vi "Test Executive.vi"(11 "Module Config":T30={"Name"="Test Executive", "Parent Q"=refnum, "Is Child?"=FALSE, "Index"=0, "Dirs"={"Root"=path "C:/MTE", "Config"=path "C:/MTE/Config", "Logs"=path "C:/MTE/Logs", "Reports"=path "C:/ATE/Reports", "App Data"=path "C:/ProgramData/Test Executive"}, "Simulate"=FALSE, "SimCtrl"=refnum}) -> ()   [LabVIEW 2018] (continued)
            n2238 = call <vilib>:"SeqMgr.Set Test Stop Criteria.vi"("Stop on Error"=w4705, "Stop on Fail"=w4706, "SeqMgr in"=w4734) -> ("SeqMgr out"=w4733:refnum<class "SeqMgr.lvclass">)  [unwired: 7 in, 1 out]
            n2239 = Build Array(w4712) -> (w4713:T31[])
            n2240 = Unbundle By Name(w4689) -> ("Opts.DisResults"=w4701:bool, "Opts.DispDetails"=w4699:bool)
            n2241 = call <vilib>:"File.Create Folder if Does Not Exist.vi"("Path"=w4698) -> ("Dup Path"=w4697:path)  [unwired: 8 in, 2 out]
            n2242 = To Variant(anything=w4713) -> (Variant=w4714:variant)
            n2243 = call <vilib>:"Q.Enqueue Task.vi"("Top of Q"=w4709, "Data1"=w4714, "Task Name"="Client - SW Items", "Q In"=w4700) -> ()  [unwired: 6 in, 2 out]
            n2244 = call <vilib>:"File.Delete Files and SubFolders in a Dir.vi"("Dir"=w4697) -> ("Dup Dir"=w4717:path)  [unwired: 9 in, 1 out]
            n2245 = Path To String(path=w4717) -> (string=w4716:string)
            n2246 = local read "Start Time"() -> (w4669:timestamp)
            n2247 = property on="Mode" class="Ring (strict)"() -> ("RingText.Text"=w4682:string)  [unwired: 2 in, 2 out]
            n2248 = local read "Default Timeout (s)"() -> (w4684:dbl)
            n2249 = local read "SN"() -> (w4740:string)
            n2250 = Bundle By Name(cluster=w4689, "DisableResults"=w4701) -> (w4665:T73)
            n2251 = Format Date/Time String(time format string (%c)="%Y_%m_%d") -> (date/time string=w4674:string)  [unwired: 2 in]
            n2252 = Select(t=1, s=w4699, f=0) -> (s? t:f=w4667:i32)
            n2253 = Format Date/Time String(time format string (%c)="%Y%m%d_%H%M%S", seconds (now)=w4669) -> (date/time string=w4672:string)  [unwired: 1 in]
            n2254 = local write "Test Status Tab Sel"(w4667) -> ()
            n2255 = local write "Test Status Tab"(w4667) -> ()
            n2256 = Number To Fractional String(number=w4684) -> (F-format string=w4742:string)  [unwired: 3 in]
            n2257 = Build Array("Mode", w4682) -> (w4680:string[])
            n2258 = Build Array("SN", w4740) -> (w4741:string[])
            n2259 = Build Array("DirSeq", w4685) -> (w4692:string[])
            n2260 = Build Array("DirCfg", w4686) -> (w4691:string[])
            n2261 = Build Array("ReportFileDir", w4716) -> (w4715:string[])
            n2262 = Build Array("Date", w4674) -> (w4676:string[])
            n2263 = Build Array("UUTDir", "") -> (w4661:string[])
            n2264 = Build Array("StartTime", w4672) -> (w4668:string[])
            n2265 = Build Array("DelaySecs", w4742) -> (w4681:string[])
            n2266 = Build Array (concatenate)(w4681, w4680, w4741, string[][] [["Failing", "0"], ["Error", "0"], ["Abort", "0"]], w4668, w4676, w4661, w4715, w4692, w4691) -> (w4735:string[][])
            n2267 = Unbundle By Name(w4665) -> ("Lists.ProcessStep"=w4663:string, "Lists.Product"=w4664:string)
            n2268 = call <vilib>:"SeqMgr.Variables - Add, Replace.vi"("Name, Value"=w4735, "Init"=TRUE, "SeqMgr in"=w4733) -> ("SeqMgr out"=w4736:refnum<class "SeqMgr.lvclass">)  [unwired: 7 in, 1 out]
            n2269 = invoke on="OperNo" class="Bool" method="Reinit To Default"() -> ()  [unwired: 3 in, 3 out]
            n2270 = invoke on="OperOK" class="Bool" method="Reinit To Default"() -> ()  [unwired: 3 in, 3 out]
            n2271 = invoke on="Prompt2_OK" class="Bool" method="Reinit To Default"() -> ()  [unwired: 3 in, 3 out]
            n2272 = call "Step Counter.Step Count Controller.vi"("Step Action"=Step_Counter.Action."Init") -> ("Step State Out"=w4732:T72)  [unwired: 8 in, 2 out]
            n2273 = Bundle By Name(cluster=w4665, "RptHdr.Test Run.ProcessStep"=w4663, "RptUUT.UUTInfo.Product"=w4664, "TimeOut(s)"="Default Timeout (s)", "SeqMgr"=w4736, "SectCtr"=w4732, "TestCanceled"=FALSE, "Data"=cluster{"FileObjs":T29[], "Meas":T38[]} {"FileObjs"=[], "Meas"=[]}) -> (w4730:T73)
            n2274 = invoke on="OperPict" class="Pict" method="Reinit To Default"() -> ()  [unwired: 3 in, 3 out]
            n2275 = property on="Operator" class="Str"("DisabledEnum"=w4724, "Text.BGColor"=w4723) -> ()  [unwired: 2 in, 2 out]
            n2276 = property on="SN" class="Str"("DisabledEnum"=w4724, "Text.BGColor"=w4723) -> ()  [unwired: 2 in, 2 out]
            n2277 = property on="Show Only Failures" class="Bool (strict)"("DisabledEnum"=T36."Disabled and Grayed Out" ("Disabled"), "Value"=FALSE ("Show Only Failures")) -> ()  [unwired: 2 in, 2 out]
            n2278 = property on="Results Table" class="Arr (strict)"("Index Values"=u32[] [0]) -> ()  [unwired: 2 in, 2 out]
          }
          frame "Test Running" {
            n2279 = Unbundle By Name(w4747) -> ("SeqMgr"=w4774:refnum<class "SeqMgr.lvclass">, "ResultState"=w4770:T63, "ResultError"=w4769:errorcluster)
            n2280 = call <vilib>:"Q.Enqueue Seq.vi"("Seq Task Name"="List Vars", "Q In"=w4751) -> ("Q Out"=w4749:refnum<queue>)  [unwired: 8 in, 1 out]
            n2281 = call <vilib>:"SeqMgr.Update Progress.vi"("error in"=w4769, "Result Info"=w4770, "SeqMgr in"=w4774) -> ("Result Info Out"=w4767:T63, "Test State"=w4771:enum32{"Idle", "Running", "Completed"}, "SeqMgr out"=w4759:refnum<class "SeqMgr.lvclass">, "New Step"=w4765:string[], "Canceled"=w4766:bool, "StepCnt"=w4748:i32)  [unwired: 2 in, 1 out]
            "Step" <- w4765
            "StepCnt" <- w4748
            n2282 = Delete From Array(array=w4765, index=0) -> (deleted portion=w4773:string, array with subset deleted=w4768:string[])  [unwired: 1 in]
            n2283 = case shown="\"Completed\"" w4771 {
              tunnel: w4773 -> [_ w4792 _]
              tunnel: w4749 -> [_ w4788 w4822]
              tunnel: ["Idle" w4790 w4826] -> w4763
              tunnel: w4767 -> [w4775 w4779 w4825]
              tunnel: w4768 -> [_ w4785 _]
              tunnel: [Event_Log.Notification_Type."Normal" ("Type") Event_Log.Notification_Type."Normal" ("Type") w4824] -> w4762
              tunnel: [Event_Log.Log_Level."Debug0" ("Level") Event_Log.Log_Level."Debug0" ("Level") Event_Log.Log_Level."Normal" ("Level")] -> w4761
              tunnel: w4748 -> [_ w4780 _]
              tunnel: w4747 -> [_ _ w4820]
              tunnel: w4746 -> [_ _ w4819]
              tunnel: [w4775 w4779 w4818] -> w4745
              frame "Idle", Default {
                # "Do Nothing"
              }
              frame "Running" {
                n2284 = To Lower Case(string=w4792) -> (all lower case string=w4794:string)
                n2285 = local read "Pause"() -> (w4791:bool)
                n2286 = Array To Spreadsheet String(delimiter (Tab)=",", array=w4785, 3:"" ("format string")) -> (spreadsheet string=w4782:string)
                n2287 = Match Pattern(string=w4794, regular expression="^sta\\.") -> (after substring=w4789:string, offset past match=w4793:i32)  [unwired: 1 in, 2 out]
                n2288 = call <vilib>:"Trim Whitespace.vi"("string"=w4782) -> ("trimmed string"=w4781:string)  [unwired: 1 in]
                n2289 = case shown="True" w4791 {
                  frame False {
                  }
                  frame True {
                    n2290 = while {
                      stop <- w4800 stop-if-true
                      n2291 = Not(x="Pause") -> (.not. x?=w4798:bool)
                      n2292 = Or(x="Inc Step", y=w4798) -> (x .or. y?=w4800:bool)
                      n2293 = Wait (ms)(milliseconds to wait=u32 100) -> ()  [unwired: 1 out]
                    }
                  }
                }
                n2294 = case shown="0, Default" w4793 {
                  tunnel: w4792 -> [w4807 w4811]
                  tunnel: w4785 -> [w4809 w4817]
                  tunnel: w4789 -> [_ _]
                  tunnel: w4788 -> [w4803 w4813]
                  frame 0, Default {
                    # "The RTN will \nCall the Test Running\nState"
                    n2295 = String Subset(string=w4807, offset (0)=4) -> (substring=w4805:string)  [unwired: 1 in]
                    n2296 = Build Array (concatenate)(w4805, w4809) -> (w4808:string[])
                    n2297 = To Variant(anything=w4808) -> (Variant=w4802:variant)
                    n2298 = call <vilib>:"Q.Enqueue Task.vi"("Data1"=w4802, "Task Name"="StaCmd", "Q In"=w4803) -> ()  [unwired: 7 in, 2 out]
                  }
                  frame -1 {
                    n2299 = To Variant(anything=w4817) -> (Variant=w4814:variant)
                    n2300 = To Variant(anything=w4811) -> (Variant=w4812:variant)
                    n2301 = call <vilib>:"Q.Enqueue Task.vi"("Data2"=w4812, "Data1"=w4814, "Task Name"="SeqCmd", "Q In"=w4813) -> ("Q Out"=w4815:refnum<queue>)  [unwired: 6 in, 1 out]
                    n2302 = call <vilib>:"Q.Enqueue Seq.vi"("Seq Task Name"="Test Running", "Q In"=w4815) -> ()  [unwired: 8 in, 2 out]
                  }
                }
                n2303 = Format Into String(format string="Test Step: Cnt_%d %s, %s", w4780, w4792, w4781) -> (resulting string=w4790:string)  [unwired: 2 in, 1 out]
              }
              frame "Completed" {
                n2304 = Flush Queue(queue=w4822) -> (queue out=w4821:refnum<queue>)  [unwired: 1 in, 2 out]
                n2305 = Unbundle By Name(w4825) -> ("State"=w4827:T1)
                n2306 = call <vilib>:"Q.Enqueue Seq.vi"("Seq Task Name"="Test Completed", "Q In"=w4821) -> ()  [unwired: 8 in, 2 out]
                n2307 = case shown="\"None\", Default" w4827 {
                  selector: w4827 -> [w4832 w4838 _ _]
                  tunnel: [w4831 w4836 w4848 w4857] -> w4826
                  tunnel: w4825 -> [w4829 w4834 w4841 w4855]
                  tunnel: [Event_Log.Notification_Type."Normal" ("Type") Event_Log.Notification_Type."Success" ("Type") Event_Log.Notification_Type."Error" ("Type") Event_Log.Notification_Type."Error" ("Type")] -> w4824
                  tunnel: w4820 -> [_ _ w4845 _]
                  tunnel: w4819 -> [_ _ w4844 _]
                  tunnel: [w4829 w4834 w4839 w4855] -> w4818
                  frame "None", Default {
                    n2308 = Format Into String(format string="Test Completed: %s" ("Seq Task Name"), w4832) -> (resulting string=w4831:string)  [unwired: 2 in, 1 out]
                  }
                  frame "Passing", "PASS" {
                    n2309 = Format Into String(format string="Test Completed: %s" ("Seq Task Name"), w4838) -> (resulting string=w4836:string)  [unwired: 2 in, 1 out]
                  }
                  frame "Failing", "FAIL" {
                    n2310 = Unbundle By Name(w4844) -> ("Cfg.Dirs.Config"=w4843:path)
                    n2311 = Unbundle By Name(w4845) -> ("Data.Meas"=w4846:T38[])
                    n2312 = call "Results.Evaluate Overall Result Based on Failure Priority.vi"("ConfigDir"=w4843, "Meas"=w4846) -> ("Change"=w4842:bool, "Result Info"=w4840:T63)  [unwired: 8 in]
                    n2313 = case shown="True" w4842 {
                      tunnel: w4841 -> [w4853 _]
                      tunnel: w4840 -> [_ w4854]
                      tunnel: [w4853 w4854] -> w4839
                      frame False {
                      }
                      frame True {
                      }
                    }
                    n2314 = Unbundle By Name(w4839) -> ("State"=w4851:T1, "Code"=w4850:i32, "Description"=w4849:string)
                    n2315 = Format Into String(format string="Test Completed: %s, %d, %s" ("Seq Task Name"), w4851, w4850, w4849) -> (resulting string=w4848:string)  [unwired: 2 in, 1 out]
                  }
                  frame "ERROR" {
                    n2316 = Unbundle By Name(w4855) -> ("State"=w4860:T1, "Code"=w4859:i32, "Description"=w4858:string)
                    n2317 = Format Into String(format string="Test Completed: %s, %d, %s" ("Seq Task Name"), w4860, w4859, w4858) -> (resulting string=w4857:string)  [unwired: 2 in, 1 out]
                  }
                }
              }
            }
            n2318 = Bundle By Name(cluster=w4747, "TestCanceled"=w4766, "SeqMgr"=w4759) -> (w4744:T73)
            n2319 = call <vilib>:"SeqMgr.Variables - Get.vi"("SeqMgr in"=w4759) -> ("Vars"=w4758:variant)  [unwired: 8 in, 2 out]
            n2320 = Get Variant Attribute(Variant=w4758) -> (names=w4754:string[], values=w4757:variant[])  [unwired: 3 in, 2 out]
            n2321 = Variant To Data(type=string[] [], Variant=w4757) -> (data=w4755:string[])  [unwired: 1 in, 1 out]
            n2322 = Build Array(w4754, w4755) -> (w4752:string[][])
            n2323 = Unbundle By Name(w4746) -> ("Log"=w4764:refnum<class "Event Notification.lvclass">)
            n2324 = Transpose 2D Array(2D array=w4752) -> (transposed array=w4753:string[][])
            n2325 = local write "Variables"(w4753) -> ()
            n2326 = call <vilib>:"Event Notification.Status Message with Error In.vi"("Log"=TRUE, "Level"=w4761, "Type"=w4762, "Message"=w4763, "Event Notification in"=w4764) -> ()  [unwired: 7 in]
            n2327 = Bundle By Name(cluster=w4744, "ResultState"=w4745) -> (w4743:T73)
          }
          frame "List Vars" {
            n2328 = Unbundle By Name(w4863) -> ("Lists.ReqVars"=w4862:bool)
            "Var Subscribe" <- w4862
            n2329 = Unbundle By Name(w4863) -> ("SeqMgr"=w4871:refnum<class "SeqMgr.lvclass">)
            n2330 = call <vilib>:"SeqMgr.Variables - Get.vi"("SeqMgr in"=w4871) -> ("Vars"=w4864:variant)  [unwired: 8 in, 2 out]
            n2331 = case shown="True" w4862 {
              tunnel: w4863 -> [_ w4876]
              tunnel: w4864 -> [_ w4873]
              frame False {
              }
              frame True {
                n2332 = Unbundle By Name(w4876) -> ("StaApp"=w4874:string)
                n2333 = call <vilib>:"Q.Enqueue Task.vi"("Data1"=w4873, "Q Name"=w4874, "Task Name"="Test Vars") -> ()  [unwired: 7 in, 2 out]
              }
            }
            n2334 = Get Variant Attribute(Variant=w4864) -> (names=w4870:string[], values=w4869:variant[])  [unwired: 3 in, 2 out]
            n2335 = Variant To Data(type=string[] [], Variant=w4869) -> (data=w4867:string[])  [unwired: 1 in, 1 out]
            n2336 = Build Array(w4870, w4867) -> (w4866:string[][])
            n2337 = Transpose 2D Array(2D array=w4866) -> (transposed array=→"Variables":string[][])
          }
          frame "Abort", "Test Abort" {
            n2338 = Unbundle By Name(w4879) -> ()  [unwired: 1 out]
            n2339 = local read "Test State"() -> (w4887:enum32{"Idle", "Running", "Completed"})
            n2340 = case shown="\"Running\"" w4887 {
              tunnel: w4879 -> [_ w4900]
              tunnel: w4880 -> [_ w4897]
              frame "Idle", Default {
              }
              frame "Running" {
                # "Return to Test Running to process the Abort"
                # "Delete timeout for \ncurrent function"
                n2341 = Unbundle By Name(w4900) -> ("Funct.Name"=w4894:string, "StaApp"=w4899:string)
                n2342 = call <vilib>:"Q.Enqueue Seq.vi"("Top of Q"=TRUE, "Seq Task Name"="Test Running", "Q In"=w4897) -> ("Q Out"=w4893:refnum<queue>)  [unwired: 7 in, 1 out]
                n2343 = local write "Abort Flag"(TRUE ("Repeat Seq")) -> ()
                n2344 = call <vilib>:"Q.Enqueue Task.vi"("Top of Q"=TRUE, "Q Name"=w4899, "Task Name"="Abort" ("Seq Task Name")) -> ()  [unwired: 7 in, 2 out]
                n2345 = call <vilib>:"Scheduler.Delete Task.vi"("Sched Name"=w4894, "Q In"=w4893) -> ()  [unwired: 8 in, 2 out]
                n2346 = for {
                  N: 5 -> [_]
                  n2347 = call "Abort.Send Abort or Done Notificaiton.vi"("Abort(T)/Done(F)"=TRUE) -> ()  [unwired: 10 in, 1 out]
                  n2348 = Wait (ms)(milliseconds to wait=u32 10) -> ()  [unwired: 1 out]
                }
              }
            }
            n2349 = local write "Repeat Seq"(FALSE ("Repeat Seq")) -> ()
            n2350 = Bundle By Name(cluster=w4879, "Funct.Seq"=0, "Funct.Name"="", "ResultState.State"=SeqMgr.Result_State_Enum."ABORT" ("State"), "ResultState.Code"=-1 ("Code"), "ResultState.Description"="Test aborted by operator.", "Repeat(s)"=-1.0) -> (w4883:T73)
            n2351 = Unbundle By Name(w4883) -> ("SeqMgr"=w4886:refnum<class "SeqMgr.lvclass">)
            n2352 = call <vilib>:"SeqMgr.Variables - Add, Replace.vi"("Name, Value"=string[][] [["Abort", "1"]] ("appended array"), "SeqMgr in"=w4886) -> ("SeqMgr out"=w4885:refnum<class "SeqMgr.lvclass">)  [unwired: 8 in, 1 out]
            n2353 = Bundle By Name(cluster=w4883, "SeqMgr"=w4885) -> (w4882:T73)
          }
          frame "Test Completed" {
            # "Clear Abort"
            n2354 = Unbundle By Name(w4915) -> ("Repeat(s)"=w4943:dbl, "Opts.NotResetSN"=w4941:bool)
            n2355 = Unbundle By Name(w4915) -> ("ResultState"=w4914:T63)
            n2356 = Unbundle By Name(w4915) -> ("Opts.DispDetails"=w4945:bool, "Opts.DisResults"=w4912:bool, "Opts.DisMetrics"=w4927:bool, "TestCanceled"=w4911:bool)
            n2357 = local write "Funct Tab"(0) -> ()
            n2358 = Unbundle By Name(w4915) -> ("StaApp"=w4918:string)
            n2359 = Unbundle By Name(w4915) -> ("PreTestCk.SNErr"=w4921:bool, "PreTestCk.NoSN"=w4924:bool, "PreTestCk.DefaultSN"=w4923:string)
            n2360 = To Variant(anything=w4914) -> (Variant=w4919:variant)
            n2361 = call <vilib>:"Q.Enqueue Task.vi"("Top of Q"=TRUE, "Data1"=w4919, "Q Name"=w4918, "Task Name"="Test Status") -> ()  [unwired: 6 in, 2 out]
            n2362 = Greater Or Equal To 0?(x=w4943) -> (x >= 0?=w4942:bool)
            n2363 = call <vilib>:"Q.Enqueue Task.vi"("Task Name"="StaTest End", "Q In"=w4934) -> ("Q Out"=w4935:refnum<queue>)  [unwired: 8 in, 1 out]
            n2364 = Or(x=w4942, y=w4941) -> (x .or. y?=w4922:bool)
            n2365 = Unbundle By Name(w4915) -> ("RptHdr.Station.SW_Config.SW_Item"=→"SW Items":T31[], "RptHdr.Test Sequence.Config.Config_Item"=→"Seq Setup":cluster{"Name":string, "Value":string}[])
            n2366 = Or(x=w4927, y=w4911) -> (x .or. y?=w4951:bool)
            n2367 = Or(x=w4922, y=w4921) -> (x .or. y?=w4920:bool)
            n2368 = case shown="True" w4945 {
              tunnel: [u32 0 w4979] -> w4913
              frame False {
              }
              frame True {
                n2369 = local read "Test Status Tab"() -> (w4975:T6)
                n2370 = To Unsigned Long Integer(number=w4975) -> (unsigned 32bit integer=w4976:u32)
                n2371 = In Range and Coerce(upper limit=u32 1, x=w4976, lower limit=u32 0) -> (coerced(x)=w4979:u32)  [unwired: 1 out]
              }
            }
            n2372 = case shown="False" w4951 {
              tunnel: w4935 -> [w4988 w4989]
              tunnel: [w4987 w4989] -> w4907
              tunnel: "Test Metrics - Add" -> [w4986 _]
              frame False {
                n2373 = call <vilib>:"Q.Enqueue Task.vi"("Task Name"=w4986, "Q In"=w4988) -> ("Q Out"=w4987:refnum<queue>)  [unwired: 8 in, 1 out]
              }
              frame True {
              }
            }
            n2374 = case shown="False" w4920 {
              tunnel: w4924 -> [w4983 _]
              tunnel: w4923 -> [w4982 _]
              frame False {
                n2375 = case shown="True" w4983 {
                  tunnel: w4982 -> [_ w4985]
                  frame False {
                    n2376 = invoke on="SN" class="Str" method="Reinit To Default"() -> ()  [unwired: 3 in, 3 out]
                    n2377 = property on="SN" class="Str"("Text.FontSize"=u32 20 ("F1")) -> ()  [unwired: 2 in, 2 out]
                  }
                  frame True {
                    n2378 = local write "SN"(w4985) -> ()
                  }
                }
              }
              frame True {
              }
            }
            n2379 = Or(x=w4912, y=w4911) -> (x .or. y?=w4910:bool)
            n2380 = call <vilib>:"Q.Enqueue Task.vi"("Task Name"="Result Comment", "Q In"=w4907) -> ("Q Out"=w4906:refnum<queue>)  [unwired: 8 in, 1 out]
            n2381 = local read "Result Status"() -> (→"Result Status 2":T2)
            n2382 = property on="SN" class="Str"("Key Focus"=TRUE) -> ()  [unwired: 2 in, 2 out]
            n2383 = case shown="False" w4910 {
              tunnel: [w4999 w5001] -> w4967
              tunnel: w4906 -> [w4999 w5000]
              frame True {
              }
              frame False {
                n2384 = call <vilib>:"Q.Enqueue Task.vi"("Task Name"="Result - Reports", "Q In"=w5000) -> ("Q Out"=w5001:refnum<queue>)  [unwired: 8 in, 1 out]
              }
            }
            n2385 = local write "Test Status Tab"(w4913) -> ()
            n2386 = local write "Test Status Tab Sel"(w4913) -> ()
            n2387 = call "Abort.Send Abort or Done Notificaiton.vi"("Abort(T)/Done(F)"=FALSE) -> ()  [unwired: 10 in, 1 out]
            n2388 = property on="State" class="Enum (strict)"() -> (error out=w4955:errorcluster, "RingText.BGColor"=w4954:u32)  [unwired: 2 in, 1 out]
            n2389 = To Variant(anything=FALSE) -> (Variant=w4968:variant)
            n2390 = Unbundle By Name(w4915) -> ("Opts.SetOpts"=w4926:bool)
            n2391 = call <vilib>:"Q.Enqueue App.vi"("Data1"=w4968, "Task Name"="Lock Test Controls", "Q In"=w4967) -> ("Q Out"=w4938:refnum<queue>)  [unwired: 7 in, 1 out]
            n2392 = Unbundle By Name(w4915) -> ("Repeat(s)"=w4930:dbl)
            n2393 = call <vilib>:"Q.Enqueue Task.vi"("Task Name"="Sta Notify", "Q In"=w4938) -> ("Q Out"=w4939:refnum<queue>)  [unwired: 8 in, 1 out]
            n2394 = property on="State" class="Enum (strict)"(error in=w4955, "RingText.BGColor"=w4954) -> ()  [unwired: 1 in, 2 out]
            n2395 = local read "Duration(s)"() -> (w4963:dbl)
            n2396 = Greater Or Equal To 0?(x=w4930) -> (x >= 0?=w4932:bool)
            n2397 = case shown="False" w4926 {
              frame False {
                n2398 = local write "Funct Tab"(u32 0) -> ()
              }
              frame True {
              }
            }
            n2399 = To Variant(anything="Init") -> (Variant=w4950:variant)
            n2400 = call <vilib>:"Q.Enqueue Seq.vi"("Data1"=w4950, "Seq Task Name"="Test Idle", "Q In"=w4939) -> ("Q Out"=w4937:refnum<queue>)  [unwired: 7 in, 1 out]
            n2401 = property on="Inc Step" class="Bool"("DisabledEnum"=T36."Disabled and Grayed Out" ("Disabled")) -> ()  [unwired: 2 in, 2 out]
            n2402 = property on="Step Run" class="Bool"("DisabledEnum"=T36."Disabled and Grayed Out" ("Disabled")) -> ()  [unwired: 2 in, 2 out]
            n2403 = case shown="True" "Repeat Seq" {
              selector: "Repeat Seq" -> [_ w4973]
              tunnel: w4932 -> [w4971 _]
              tunnel: [w4971 w4973] -> w4931
              tunnel: w4930 -> [w4970 _]
              tunnel: [w4970 w4972] -> w4929
              tunnel: "RepeatInt(s)" -> [_ w4972]
              frame False {
              }
              frame True {
              }
            }
            n2404 = local read "SN Rslt"() -> (w4944:string)
            n2405 = stacked-sequence {
              frame #0 {
                n2406 = local write "Test Ctrl Tab"(enum32{"Idle", "Running", "Completed"}."Idle" ("Test Ctrl Tab")) -> ()
              }
              frame #1 {
                n2407 = property on="Start" class="Bool"("Key Focus"=TRUE) -> ()  [unwired: 2 in, 2 out]
              }
            }
            n2408 = Bundle By Name(cluster=w4915, "RptHdr.Test Run.Duration(s)"=w4963) -> (w4964:T73)
            n2409 = case shown="True" w4931 {
              tunnel: "Repeat Sequence" ("Sched Name") -> [_ w4998]
              tunnel: w4929 -> [_ w4997]
              tunnel: w4937 -> [_ w4996]
              tunnel: w4944 -> [_ w4990]
              frame False {
              }
              frame True {
                w4992 = TRUE ("Visible")
                n2410 = To Variant(anything=w4990) -> (Variant=w4991:variant)
                n2411 = call <vilib>:"Scheduler.AddTask.vi"("Data1"=w4991, "Interval(s)"=w4997, "Task Name"=w4998, "Sched Name"=w4998, "Q In"=w4996) -> ("Q Out"=w4995:refnum<queue>)  [unwired: 5 in, 1 out]
                n2412 = property on="Repeat Notificaiton" class="Str"("Visible"=w4992) -> ()  [unwired: 2 in, 2 out]
                n2413 = property on="Kill AutoLnch" class="Bool"("Visible"=w4992) -> ()  [unwired: 2 in, 2 out]
                n2414 = call <vilib>:"Q.Enqueue Task.vi"("Top of Q"=TRUE, "Task Name"="Repeat Notification" ("Sched Name"), "Q In"=w4995) -> ()  [unwired: 7 in, 2 out]
              }
            }
            n2415 = property on="Show Only Failures" class="Bool (strict)"("DisabledEnum"=T36."Enabled" ("Disabled")) -> ()  [unwired: 2 in, 2 out]
            "Test State" <- enum32{"Idle", "Running", "Completed"}."Completed" ("Test State")
          }
          frame "Test Reset" {
            w5008 = picture data[5B] ("Rigth Image")
            w5015 = FALSE
            w5028 = u32 16448250
            w5031 = T36."Enabled" ("Disabled")
            # "Clear Abort Notificaiton"
            # "Clear data to prepare for a new test"
            n2416 = Obtain Notifier(name (unnamed)="Abort", notification data type=w5015) -> (notifier out=w5019:refnum<notifier>, error out=w5018:errorcluster)  [unwired: 2 in, 1 out]
            n2417 = call <vilib>:"Scheduler.Delete Task.vi"("Sched Name"="Repeat Sequence", "Q In"=w5034) -> ("Q Out"=w5012:refnum<queue>)  [unwired: 8 in, 1 out]
            n2418 = invoke on="SN Rslt" class="Str" method="Reinit To Default"() -> ()  [unwired: 3 in, 3 out]
            n2419 = Unbundle By Name(w5027) -> ("Log"=w5026:refnum<class "Event Notification.lvclass">)
            n2420 = Send Notification(notification=w5015, notifier=w5019, error in (no error)=w5018) -> (notifier out=w5016:refnum<notifier>, error out=w5017:errorcluster)
            n2421 = call <vilib>:"Q.Enqueue Task.vi"("Task Name"="Sta Test Reset", "Q In"=w5012) -> ("Q Out"=w5011:refnum<queue>)  [unwired: 8 in, 1 out]
            n2422 = call <vilib>:"Event Notification.Status Message.vi"("Display"=TRUE, "Level"=Event_Log.Log_Level."Normal", "Message"="Idle", "Event Notification in"=w5026) -> ()  [unwired: 8 in]
            n2423 = Release Notifier(notifier=w5016, force destroy? (F)=TRUE, error in (no error)=w5017) -> ()  [unwired: 3 out]
            n2424 = To Variant(anything="Init") -> (Variant=w5040:variant)
            n2425 = call <vilib>:"Q.Enqueue Seq.vi"("Data1"=w5040, "Seq Task Name"="Test Idle", "Q In"=w5011) -> ()  [unwired: 7 in, 2 out]
            n2426 = property on="Kill AutoLnch" class="Bool"("Visible"=FALSE) -> ()  [unwired: 2 in, 2 out]
            n2427 = property on="Repeat Notificaiton" class="Str"("Visible"=FALSE) -> ()  [unwired: 2 in, 2 out]
            n2428 = Unbundle By Name(w5007) -> ("SeqMgr"=w5044:refnum<class "SeqMgr.lvclass">, "Opts.NotResetSN"=w5020:bool, "Repeat(s)"=w5022:dbl)
            n2429 = local write "Test State"(enum32{"Idle", "Running", "Completed"}."Idle" ("Test State")) -> ()
            n2430 = invoke on="Duration(HH:MM:SS)" class="Str" method="Reinit To Default"() -> ()  [unwired: 3 in, 3 out]
            n2431 = Unbundle By Name(w5007) -> ("PreTestCk.NoSN"=w5006:bool, "PreTestCk.DefaultSN"=w5005:string, "PreTestCk.SeqEn"=w5003:T36)
            n2432 = Greater Or Equal To 0?(x=w5022) -> (x >= 0?=w5023:bool)
            n2433 = property on="SN" class="Str"("Key Focus"=TRUE) -> ()  [unwired: 2 in, 2 out]
            n2434 = Or(x=w5020, y=w5023) -> (x .or. y?=w5021:bool)
            n2435 = case shown="False" w5021 {
              tunnel: w5006 -> [w5049 _]
              tunnel: w5005 -> [w5048 _]
              frame False {
                n2436 = case shown="True" w5049 {
                  tunnel: w5048 -> [_ w5051]
                  frame False {
                    n2437 = invoke on="SN" class="Str" method="Reinit To Default"() -> ()  [unwired: 3 in, 3 out]
                    n2438 = property on="SN" class="Str"("Text.FontSize"=u32 20 ("F1")) -> ()  [unwired: 2 in, 2 out]
                  }
                  frame True {
                    n2439 = local write "SN"(w5051) -> ()
                  }
                }
              }
              frame True {
              }
            }
            n2440 = property on="Operator" class="Str"("DisabledEnum"=w5031, "Text.BGColor"=w5028) -> ()  [unwired: 2 in, 2 out]
            n2441 = call <vilib>:"SeqMgr.Test Reset.vi"("SeqMgr in"=w5044) -> ("SeqMgr out"=w5045:refnum<class "SeqMgr.lvclass">)  [unwired: 9 in, 1 out]
            n2442 = property on="SN" class="Str"("DisabledEnum"=w5031, "Text.BGColor"=w5028) -> ()  [unwired: 2 in, 2 out]
            n2443 = property on="Sequence" class="Ring (strict)"("DisabledEnum"=w5003) -> ()  [unwired: 2 in, 2 out]
            n2444 = property on="Results Table" class="Arr (strict)"("Index Values"=u32[] [0]) -> ()  [unwired: 2 in, 2 out]
            n2445 = Bundle By Name(cluster=w5007, "SeqMgr"=w5045) -> (w5043:T73)
            n2446 = invoke on="OperPrompt" class="Str" method="Reinit To Default"() -> ()  [unwired: 3 in, 3 out]
            n2447 = invoke on="Abort Flag" class="Bool (strict)" method="Reinit To Default"() -> ()  [unwired: 3 in, 3 out]
            n2448 = invoke on="Results Table" class="Arr (strict)" method="Reinit To Default"() -> ()  [unwired: 3 in, 3 out]
            n2449 = invoke on="OperPict" class="Pict" method="Reinit To Default"() -> ()  [unwired: 3 in, 3 out]
            n2450 = invoke on="Variables" class="Arr (strict)" method="Reinit To Default"() -> ()  [unwired: 3 in, 3 out]
            n2451 = invoke on="OperNo" class="Bool" method="Reinit To Default"() -> ()  [unwired: 3 in, 3 out]
            n2452 = invoke on="OperOK" class="Bool" method="Reinit To Default"() -> ()  [unwired: 3 in, 3 out]
            n2453 = invoke on="Prompt2_OK" class="Bool" method="Reinit To Default"() -> ()  [unwired: 3 in, 3 out]
            n2454 = invoke on="Progress 2" class="Slide (strict)" method="Reinit To Default"() -> ()  [unwired: 3 in, 3 out]
            n2455 = Bundle By Name(cluster=w5043, "RptHdr.Test Run"=T48 {"Operator"="", "Start Time"=timestamp(0 s since 1904-01-01), "Duration(s)"=0.0, "Mode"="", "Comment"="", "ProcessStep"=""} ("RptHdrInfo.Test Run"), "RptHdr.Test Sequence"=T49 {"Name"="", "Config"={"Config_Item"=[]}} ("RptHdrInfo.Test Sequence"), "RptUUT"=T50 {"Position"="", "Result"={"Result"=enum."Pass", "Code"=0, "Description"=""}, "Measurements"={"Measurement"=[]}, "UUTInfo"={"Product"="", "Desc"="", "PN"="", "SN"="", "Lot"="", "DateCode"="", "AltID"="", "Revision"="", "Properties"={"Property"=[]}}} ("RptUUTInfo"), "Data"=cluster{"FileObjs":T29[], "Meas":T38[]} {"FileObjs"=[], "Meas"=[]}) -> (w5046:T73)
            n2456 = local write "Rigth Image"(w5008) -> ()
            n2457 = local write "Left Image"(w5008) -> ()
            n2458 = invoke on="UUT Properties" class="Arr (strict)" method="Reinit To Default"() -> ()  [unwired: 3 in, 3 out]
            n2459 = invoke on="File Data Objs" class="Arr (strict)" method="Reinit To Default"() -> ()  [unwired: 3 in, 3 out]
            n2460 = invoke on="SeqPN" class="Str" method="Reinit To Default"() -> ()  [unwired: 3 in, 3 out]
            n2461 = invoke on="SeqVer" class="Str" method="Reinit To Default"() -> ()  [unwired: 3 in, 3 out]
            n2462 = invoke on="Seq Setup" class="Arr (strict)" method="Reinit To Default"() -> ()  [unwired: 3 in, 3 out]
            n2463 = invoke on="SeqName" class="Str" method="Reinit To Default"() -> ()  [unwired: 3 in, 3 out]
            "Test Ctrl Tab" <- enum32{"Idle", "Running", "Completed"}."Idle" ("Test Ctrl Tab")
          }
        }
      }
      frame "Function" {
        n2464 = case shown="Default" w5059 {
          tunnel: w5063 -> [w5066]
          tunnel: w5062 -> [w5067]
          tunnel: [w5066] -> w5061
          tunnel: [w5067] -> w5060
          tunnel: w5058 -> [_]
          tunnel: w5057 -> [_]
          tunnel: w5056 -> [w5064]
          tunnel: w5054 -> [_]
          tunnel: [w5064] -> w5053
          tunnel: [variant] -> w5052
          frame Default {
            # "Do nothing.  The sender of the command will report an error (timeout or incorrect data)."
          }
        }
        n2465 = call <vilib>:"Q.Return Function Data.vi"("error in"=w5053, "Data2"=w5054, "Ret Data"=w5052) -> ("error out"=w5055:errorcluster)  [unwired: 8 in]
      }
      frame "App" {
        n2466 = case shown="\"Set Logging Level\"" w5070 {
          tunnel: w5076 -> [w5078 w5084 w5098 w5128 w5212 w5223 w5240]
          tunnel: [w5078 w5084 w5098 w5128 w5211 w5225 w5240] -> w5075
          tunnel: w5074 -> [w5077 w5080 w5094 w5131 w5213 w5224 w5239]
          tunnel: [w5077 w5080 w5094 w5130 w5213 w5224 w5239] -> w5073
          tunnel: w5072 -> [_ _ w5097 w5134 _ w5226 _]
          tunnel: [_ _ errorcluster {"status"=FALSE, "code"=0, "source"=""} ("error constant") _ _ _ _] -> w5071
          tunnel: w5069 -> [_ w5089 _ _ _ w5219 _]
          tunnel: w5068 -> [_ _ _ w5129 _ _ _]
          frame Default {
          }
          frame "Initialization Done" {
            # "Unlock Controls"
            # "Set Status"
            n2467 = Unbundle By Name(w5084) -> ("Log"=w5083:refnum<class "Event Notification.lvclass">)
            n2468 = call <vilib>:"Event Notification.Status Message.vi"("Log"=TRUE, "Message"="Initialization Done, Going to Idle", "Event Notification in"=w5083) -> ()  [unwired: 9 in]
            n2469 = To Variant(anything=FALSE) -> (Variant=w5092:variant)
            n2470 = call <vilib>:"Q.Enqueue App.vi"("Data1"=w5092, "Task Name"="Lock Test Controls", "Q In"=w5089) -> ("Q Out"=w5087:refnum<queue>)  [unwired: 7 in, 1 out]
            n2471 = Unbundle By Name(w5080) -> ("CfgFilePaths"=→"CfgFilePaths":T67)
            n2472 = To Variant(anything="Init") -> (Variant=w5085:variant)
            n2473 = call <vilib>:"Q.Enqueue Seq.vi"("Data1"=w5085, "Seq Task Name"="Test Idle", "Q In"=w5087) -> ()  [unwired: 7 in, 2 out]
          }
          frame "Lock Test Controls" {
            n2474 = Variant To Data(type=FALSE, Variant=w5097) -> (data=w5095:bool, error out=w5096:errorcluster)  [unwired: 1 in]
            n2475 = case shown="No Error" w5096 {
              selector: w5096 -> [_ w5127]
              tunnel: w5095 -> [w5111 _]
              tunnel: [_ w5127] -> _
              tunnel: w5094 -> [w5101 _]
              frame No Error {
                n2476 = case shown="True" w5111 {
                  tunnel: [T36."Enabled" ("Disabled") w5123] -> w5100
                  tunnel: [T36."Enabled" ("Disabled") T36."Disabled" ("Disabled")] -> w5102
                  tunnel: [TRUE ("Enable") FALSE ("Enable")] -> w5110
                  tunnel: [_ TRUE ("Enable")] -> w5104
                  tunnel: [w5117 w5123] -> _
                  tunnel: w5101 -> [w5119 _]
                  frame False {
                    n2477 = Unbundle By Name(w5119) -> ("Opts.GenRpt"=w5118:bool)
                    n2478 = Select(t=T36."Enabled" ("Disabled"), s=w5118, f=T36."Disabled and Grayed Out" ("Disabled")) -> (s? t:f=w5117:T36)
                  }
                  frame True {
                    w5123 = T36."Disabled and Grayed Out" ("Disabled")
                  }
                }
                n2479 = Unbundle By Name(w5101) -> ("App.Child Modules"=w5107:cluster{"VI Ref":refnum<vi>, "Name":string}[])
                n2480 = case shown="True" FALSE ("Enable") {
                  tunnel: w5110 -> [_ w5112]
                  frame False {
                  }
                  frame True {
                    n2481 = Current VI's Menubar() -> (w5113:refnum<k9>)
                    n2482 = call <vilib>:"Menu.Enable Item.vi"("Enable"=w5112, "Tag"="Config", "Menu Ref"=w5113) -> ()  [unwired: 7 in, 2 out]
                  }
                }
                n2483 = property on="Filter" class="Str"("DisabledEnum"=w5100) -> ()  [unwired: 2 in, 2 out]
                n2484 = property on="Test Reset" class="Bool"("DisabledEnum"=w5100) -> ()  [unwired: 2 in, 2 out]
                n2485 = Index Array(array=w5107) -> (element=w5106:cluster{"VI Ref":refnum<vi>, "Name":string})  [unwired: 1 in]
                n2486 = Unbundle By Name(w5106) -> ("Name"=w5105:string)
                n2487 = property on="Mode" class="Ring (strict)"("DisabledEnum"=w5102) -> ()  [unwired: 2 in, 2 out]
                n2488 = To Variant(anything=w5104) -> (Variant=w5109:variant)
                n2489 = call <vilib>:"Q.Enqueue App.vi"("Data1"=w5109, "Q Name"=w5105, "Task Name"="Lock Test Controls") -> ()  [unwired: 7 in, 2 out]
              }
              frame Error {
              }
            }
          }
          frame "Health Status" {
            n2490 = Variant To Data(type=TestExec.Health_State_Command."Clear Errors" ("Health State Cmd"), Variant=w5134) -> (data=w5132:T37)  [unwired: 1 in, 1 out]
            n2491 = case shown="\"Set Warning\"" w5132 {
              tunnel: w5131 -> [w5139 w5147 w5156 w5176 w5193 w5204]
              tunnel: [w5139 w5146 w5155 w5177 w5194 w5203] -> w5130
              tunnel: w5129 -> [_ _ _ w5175 w5192 _]
              tunnel: w5128 -> [_ _ _ w5166 _ _]
              frame "Update", Default {
                n2492 = control-ref of="Go to Health Details"() -> (w5135:refnum<vi>)
                n2493 = control-ref of="Warnings"() -> (w5137:refnum<vi>)
                n2494 = control-ref of="Errors"() -> (w5136:refnum<vi>)
                n2495 = control-ref of="Health OK"() -> (w5138:refnum<vi>)
                n2496 = call "TestExec.Health Indicator State Controller.vi"("Go to Details"=w5135, "Errors Cntr"=w5136, "Warnings Cntr"=w5137, "Health Bool"=w5138) -> ()  [unwired: 8 in]
              }
              frame "Clear All" {
                n2497 = invoke on="Error List" class="Arr (strict)" method="Reinit To Default"() -> (error out=w5143:errorcluster)  [unwired: 3 in, 2 out]
                n2498 = invoke on="Warning List" class="Arr (strict)" method="Reinit To Default"() -> (error out=w5142:errorcluster)  [unwired: 3 in, 2 out]
                n2499 = invoke on="Warnings" class="DigNum (strict)" method="Reinit To Default"(error in=w5142) -> (error out=w5140:errorcluster)  [unwired: 2 in, 2 out]
                n2500 = invoke on="Errors" class="DigNum (strict)" method="Reinit To Default"(error in=w5143) -> (error out=w5141:errorcluster)  [unwired: 2 in, 2 out]
                n2501 = flat-sequence {
                  tunnel: w5141 -> [_]
                  tunnel: w5140 -> [_]
                  frame #0 {
                    n2502 = control-ref of="Go to Health Details"() -> (w5148:refnum<vi>)
                    n2503 = control-ref of="Warnings"() -> (w5150:refnum<vi>)
                    n2504 = control-ref of="Errors"() -> (w5149:refnum<vi>)
                    n2505 = control-ref of="Health OK"() -> (w5151:refnum<vi>)
                    n2506 = call "TestExec.Health Indicator State Controller.vi"("Go to Details"=w5148, "Errors Cntr"=w5149, "Warnings Cntr"=w5150, "Health Bool"=w5151) -> ()  [unwired: 8 in]
                  }
                }
                n2507 = Bundle By Name(cluster=w5147, "Health.Warnings"=0, "Health.Errors"=0) -> (w5146:T73)
              }
              frame "Clear Errors" {
                n2508 = invoke on="Error List" class="Arr (strict)" method="Reinit To Default"() -> (error out=w5153:errorcluster)  [unwired: 3 in, 2 out]
                n2509 = invoke on="Errors" class="DigNum (strict)" method="Reinit To Default"(error in=w5153) -> (error out=w5152:errorcluster)  [unwired: 2 in, 2 out]
                n2510 = flat-sequence {
                  tunnel: w5152 -> [_]
                  frame #0 {
                    n2511 = control-ref of="Go to Health Details"() -> (w5157:refnum<vi>)
                    n2512 = control-ref of="Warnings"() -> (w5159:refnum<vi>)
                    n2513 = control-ref of="Errors"() -> (w5158:refnum<vi>)
                    n2514 = control-ref of="Health OK"() -> (w5160:refnum<vi>)
                    n2515 = call "TestExec.Health Indicator State Controller.vi"("Go to Details"=w5157, "Errors Cntr"=w5158, "Warnings Cntr"=w5159, "Health Bool"=w5160) -> ()  [unwired: 8 in]
                  }
                }
                n2516 = Bundle By Name(cluster=w5156, "Health.Errors"=0) -> (w5155:T73)
              }
              frame "Set Warning" {
                n2517 = Unbundle By Name(w5166) -> ("Log"=w5165:refnum<class "Event Notification.lvclass">)
                n2518 = Variant To Data(type=errorcluster {"status"=FALSE, "code"=0, "source"=""} ("error constant"), Variant=w5175) -> (data=w5172:errorcluster)  [unwired: 1 in, 1 out]
                n2519 = Unbundle By Name(w5172) -> ("code"=w5171:i32, "source"=w5161:string)
                n2520 = Bundle By Name(cluster=T10 {"Code"=0, "Desc"="", "First"=timestamp(0 s since 1904-01-01), "Last"=timestamp(0 s since 1904-01-01), "Count"=0} ("Warning"), "Code"=w5171, "Desc"=w5161) -> (w5168:T10)
                n2521 = local read "Warning List"() -> (w5170:T10[])
                n2522 = Concatenate Strings("Warning:", w5161) -> (w5163:string)
                n2523 = call "TestExec.Add Warning, Skip if redundant.vi"("Warning"=w5168, "Warning List"=w5170) -> ("Count"=w5167:i32, "Warning List Out"=→"Warning List":T10[])  [unwired: 8 in]
                n2524 = call <vilib>:"Event Notification.Status Message.vi"("Log"=TRUE, "Message"=w5163, "Event Notification in"=w5165) -> ()  [unwired: 9 in]
                n2525 = Bundle By Name(cluster=w5176, "Health.Warnings"=w5167) -> (w5177:T73)
                n2526 = flat-sequence {
                  tunnel: w5167 -> [w5178]
                  frame #0 {
                    "Warnings" <- w5178
                  }
                  frame #1 {
                    n2527 = control-ref of="Go to Health Details"() -> (w5179:refnum<vi>)
                    n2528 = control-ref of="Warnings"() -> (w5181:refnum<vi>)
                    n2529 = control-ref of="Errors"() -> (w5180:refnum<vi>)
                    n2530 = control-ref of="Health OK"() -> (w5182:refnum<vi>)
                    n2531 = call "TestExec.Health Indicator State Controller.vi"("Go to Details"=w5179, "Errors Cntr"=w5180, "Warnings Cntr"=w5181, "Health Bool"=w5182) -> ()  [unwired: 8 in]
                  }
                }
              }
              frame "Set Error" {
                n2532 = Variant To Data(type=errorcluster {"status"=FALSE, "code"=0, "source"=""} ("error constant"), Variant=w5192) -> (data=w5188:errorcluster)  [unwired: 1 in, 1 out]
                n2533 = Unbundle By Name(w5188) -> ("code"=w5190:i32, "source"=w5189:string)
                n2534 = local read "Error List"() -> (w5186:T11[])
                n2535 = Bundle By Name(cluster=T11 {"Code"=0, "Desc"="", "First"=timestamp(0 s since 1904-01-01), "Last"=timestamp(0 s since 1904-01-01), "Count"=0} ("Error"), "Code"=w5190, "Desc"=w5189) -> (w5183:T11)
                n2536 = call "TestExec.Add Error, Skip if redundant.vi"("Error"=w5183, "Error List"=w5186) -> ("Count"=w5184:i32, "Error List Out"=→"Error List":T11[])  [unwired: 8 in]
                n2537 = flat-sequence {
                  tunnel: w5184 -> [w5195]
                  frame #0 {
                    "Errors" <- w5195
                  }
                  frame #1 {
                    n2538 = control-ref of="Warnings"() -> (w5196:refnum<vi>)
                    n2539 = control-ref of="Go to Health Details"() -> (w5197:refnum<vi>)
                    n2540 = control-ref of="Errors"() -> (w5198:refnum<vi>)
                    n2541 = control-ref of="Health OK"() -> (w5199:refnum<vi>)
                    n2542 = call "TestExec.Health Indicator State Controller.vi"("Go to Details"=w5197, "Errors Cntr"=w5198, "Warnings Cntr"=w5196, "Health Bool"=w5199) -> ()  [unwired: 8 in]
                  }
                }
                n2543 = Bundle By Name(cluster=w5193, "Health.Errors"=w5184) -> (w5194:T73)
              }
              frame "Clear Warnings" {
                n2544 = invoke on="Warning List" class="Arr (strict)" method="Reinit To Default"() -> (error out=w5201:errorcluster)  [unwired: 3 in, 2 out]
                n2545 = invoke on="Warnings" class="DigNum (strict)" method="Reinit To Default"(error in=w5201) -> (error out=w5200:errorcluster)  [unwired: 2 in, 2 out]
                n2546 = flat-sequence {
                  tunnel: w5200 -> [_]
                  frame #0 {
                    n2547 = control-ref of="Go to Health Details"() -> (w5205:refnum<vi>)
                    n2548 = control-ref of="Warnings"() -> (w5207:refnum<vi>)
                    n2549 = control-ref of="Errors"() -> (w5206:refnum<vi>)
                    n2550 = control-ref of="Health OK"() -> (w5208:refnum<vi>)
                    n2551 = call "TestExec.Health Indicator State Controller.vi"("Go to Details"=w5205, "Errors Cntr"=w5206, "Warnings Cntr"=w5207, "Health Bool"=w5208) -> ()  [unwired: 8 in]
                  }
                }
                n2552 = Bundle By Name(cluster=w5204, "Health.Warnings"=0) -> (w5203:T73)
              }
            }
          }
          frame "Set Logging Level" {
            n2553 = Unbundle By Name(w5212) -> ("Log"=w5214:refnum<class "Event Notification.lvclass">)
            n2554 = Format Into String(format string="Logging Level Set to %s", "Log Level") -> (resulting string=w5216:string)  [unwired: 2 in, 1 out]
            n2555 = call <vilib>:"Event Notification.Status Message.vi"("Log"=TRUE, "Level"=Event_Log.Log_Level."Normal", "Message"=w5216, "Event Notification in"=w5214) -> ()  [unwired: 8 in]
            n2556 = call <vilib>:"Event Notification.Set Logging Level.vi"("Log Level"="Log Level", "Event Notification in"=w5214) -> ("Event Notification out"=w5215:refnum<class "Event Notification.lvclass">)  [unwired: 9 in]
            n2557 = Bundle By Name(cluster=w5212, "Log"=w5215) -> (w5211:T33)
          }
          frame "Simulate" {
            # "Forward Simulate state to child modules"
            n2558 = Variant To Data(type=FALSE, Variant=w5226) -> (data=w5221:bool)  [unwired: 1 in, 1 out]
            n2559 = Unbundle By Name(w5223) -> ("Cfg.Is Child?"=w5228:bool, "Cfg.Dirs.Config"=w5229:path)
            n2560 = Unbundle By Name(w5223) -> ("Cfg.Simulate"=w5222:bool)
            n2561 = Not Equal?(x=w5222, y=w5221) -> (x != y?=w5220:bool)
            n2562 = case shown="False" w5228 {
              tunnel: w5229 -> [w5234 _]
              tunnel: w5221 -> [w5233 _]
              frame False {
                n2563 = call <vilib>:"Config.Simulate.Set.vi"("Simulate"=w5233, "Config Folder"=w5234) -> ()  [unwired: 9 in, 1 out]
              }
              frame True {
              }
            }
            n2564 = case shown="True" w5220 {
              tunnel: w5219 -> [_ w5232]
              frame False {
              }
              frame True {
                n2565 = call <vilib>:"Q.Enqueue Reset.vi"("Q In"=w5232) -> ()  [unwired: 9 in, 2 out]
              }
            }
            n2566 = Bundle By Name(cluster=w5223, "Cfg.Simulate"=w5221) -> (w5225:T33)
            n2567 = property on="Simulate Indication" class="Str"("Visible"=w5221) -> ()  [unwired: 2 in, 2 out]
            n2568 = Unbundle By Name(w5224) -> ("App.Child Modules"=w5231:cluster{"VI Ref":refnum<vi>, "Name":string}[])
            n2569 = To Variant(anything=w5221) -> (Variant=w5230:variant)
            n2570 = for {
              tunnel: w5231 -> [w5238] mode=indexing
              tunnel: w5230 -> [w5235]
              n2571 = Unbundle By Name(w5238) -> ("Name"=w5237:string)
              n2572 = call <vilib>:"Q.Enqueue Task.vi"("Data1"=w5235, "Q Name"=w5237, "Task Name"="Simulate") -> ()  [unwired: 7 in, 2 out]
            }
          }
          frame "Simulate Fwd" {
            # "Forward Simulate state to child modules"
            n2573 = Unbundle By Name(w5240) -> ("Cfg.Simulate"=w5241:bool)
            n2574 = Unbundle By Name(w5239) -> ("App.Child Modules"=w5243:cluster{"VI Ref":refnum<vi>, "Name":string}[])
            n2575 = To Variant(anything=w5241) -> (Variant=w5242:variant)
            n2576 = for {
              tunnel: w5243 -> [w5247] mode=indexing
              tunnel: w5242 -> [w5244]
              n2577 = Unbundle By Name(w5247) -> ("Name"=w5246:string)
              n2578 = call <vilib>:"Q.Enqueue Task.vi"("Data1"=w5244, "Q Name"=w5246, "Task Name"="Simulate") -> ()  [unwired: 7 in, 2 out]
            }
          }
        }
      }
      frame "Error", Default {
        n2579 = case shown="\"Error\"" w5254 {
          selector: w5254 -> [_ w5277]
          tunnel: [_ w5278] -> w5255
          tunnel: w5253 -> [w5269 _]
          tunnel: w5252 -> [w5267 _]
          tunnel: w5251 -> [w5268 _]
          tunnel: w5250 -> [w5266 _]
          tunnel: w5249 -> [w5265 w5276]
          tunnel: [w5264 w5276] -> w5248
          tunnel: [w5257 _] -> _
          frame "Error" {
            n2580 = case shown="Default" w5268 {
              tunnel: w5269 -> [_ w5275]
              tunnel: w5267 -> [w5271 _]
              tunnel: [w5271 w5273] -> w5259
              tunnel: w5266 -> [w5270 w5272]
              tunnel: [w5270 w5272] -> w5260
              frame Default {
              }
              frame "Error" {
                n2581 = Variant To Data(type=errorcluster {"status"=FALSE, "code"=0, "source"=""} ("error constant"), Variant=w5275) -> (data=w5273:errorcluster)  [unwired: 1 in, 1 out]
              }
            }
            n2582 = Bundle By Name(cluster=w5265, "ResultError"=w5259) -> (w5264:T73)
            n2583 = call <vilib>:"Event Log.Record Event.vi"("error in"=w5259) -> ("error out"=w5257:errorcluster)  [unwired: 10 in]
            n2584 = To Variant(anything=TestExec.Health_State_Command."Set Error" ("Health State Cmd")) -> (Variant=w5263:variant)
            n2585 = To Variant(anything=w5259) -> (Variant=w5258:variant)
            n2586 = call <vilib>:"Q.Enqueue App.vi"("Data2"=w5258, "Data1"=w5263, "Task Name"="Health Status", "Q In"=w5260) -> ()  [unwired: 6 in, 2 out]
          }
          frame Default {
            n2587 = Concatenate Strings("Undefined State: \"", w5277, "\".") -> (w5279:string)
            n2588 = Bundle By Name(cluster=errorcluster {"status"=TRUE, "code"=-5000, "source"=""} ("error constant"), "source"=w5279) -> (w5278:errorcluster)
          }
        }
      }
      frame "Exit" {
        n2589 = stacked-sequence {
          tunnel: w5285 -> [_ w5298 _ _ _]
          tunnel: [errorcluster {"status"=FALSE, "code"=0, "source"=""} ("error constant") _ _ _ _] -> w5284
          tunnel: w5283 -> [_ _ w5307 _ _]
          tunnel: [_ _ _ _ w5324] -> _
          tunnel: [_ _ w5305 _ _] -> _
          tunnel: [_ _ w5303 _ _] -> _
          frame #0 {
            # "Close connection to instruments"
            n2590 = property on="PLC" class="Bool (strict)"() -> ("Visible"=w5290:bool)  [unwired: 2 in, 2 out]
            n2591 = case shown="True" w5290 {
              frame False {
              }
              frame True {
                n2592 = call <vilib>:"Q.Enqueue Exit.vi"("Q Name"="PLC") -> ("error out"=w5292:errorcluster)  [unwired: 9 in, 1 out]
                n2593 = call <vilib>:"Clear Errors.vi"("error in (no error)"=w5292) -> ()  [unwired: 5 in, 2 out]
              }
            }
            n2594 = call <vilib>:"Q.Enqueue Exit.vi"("Q Name"="Wiggler") -> ("error out"=w5288:errorcluster)  [unwired: 9 in, 1 out]
            n2595 = call <vilib>:"Clear Errors.vi"("error in (no error)"=w5288) -> ()  [unwired: 5 in, 2 out]
          }
          frame #1 {
            # "Send Exit command to child modules"
            n2596 = Unbundle By Name(w5298) -> ("App.Child Modules"=w5299:cluster{"VI Ref":refnum<vi>, "Name":string}[])
            n2597 = Unbundle By Name(w5298) -> ("StaApp"=w5294:string)
            n2598 = for {
              tunnel: w5299 -> [w5302] mode=indexing
              tunnel: [w5300] -> w5297
              n2599 = Unbundle By Name(w5302) -> ("Name"=w5301:string)
              n2600 = call <vilib>:"Q.Enqueue Exit.vi"("Q Name"=w5301) -> ("error out"=w5300:errorcluster)  [unwired: 9 in, 1 out]
            }
            n2601 = call <vilib>:"Clear Errors.vi"("error in (no error)"=w5297) -> ("error out"=w5296:errorcluster)  [unwired: 5 in, 1 out]
            n2602 = call <vilib>:"Q.Enqueue Exit.vi"("Q Name"=w5294, "Error In"=w5296) -> ("error out"=w5295:errorcluster)  [unwired: 8 in, 1 out]
            n2603 = call <vilib>:"Clear Errors.vi"("error in (no error)"=w5295) -> ()  [unwired: 5 in, 2 out]
          }
          frame #2 {
            n2604 = Unbundle By Name(w5307) -> ("Cfg.Dirs.Logs"=w5309:path)
            n2605 = call "TestExec.Test Metric Add_Get.vi"("Log Dir"=w5309, "Action"=TestExec.Test_Metric_Action_Selector."Save") -> ()  [unwired: 8 in, 2 out]
            n2606 = call <vilib>:"Q.Enqueue Exit.vi"("Q Name"="ArchiveMover" ("Control Q")) -> ("error out"=w5305:errorcluster)  [unwired: 9 in, 1 out]
            n2607 = call <vilib>:"Q.Enqueue Exit.vi"("Q Name"="FileRotate") -> ("error out"=w5303:errorcluster)  [unwired: 9 in, 1 out]
          }
          frame #3 {
            w5315 = u32 16448250
            n2608 = invoke on="Error List" class="Arr (strict)" method="Reinit To Default"() -> ()  [unwired: 3 in, 3 out]
            n2609 = invoke on="Warning List" class="Arr (strict)" method="Reinit To Default"() -> ()  [unwired: 3 in, 3 out]
            n2610 = invoke on="Warnings" class="DigNum (strict)" method="Reinit To Default"() -> (error out=w5313:errorcluster)  [unwired: 3 in, 2 out]
            n2611 = invoke on="Errors" class="DigNum (strict)" method="Reinit To Default"() -> (error out=w5314:errorcluster)  [unwired: 3 in, 2 out]
            n2612 = property on="Position" class="Str"("Visible"=TRUE) -> ()  [unwired: 2 in, 2 out]
            n2613 = flat-sequence {
              tunnel: w5314 -> [_]
              tunnel: w5313 -> [_]
              frame #0 {
                n2614 = control-ref of="Go to Health Details"() -> (w5317:refnum<vi>)
                n2615 = control-ref of="Warnings"() -> (w5319:refnum<vi>)
                n2616 = control-ref of="Errors"() -> (w5318:refnum<vi>)
                n2617 = control-ref of="Health OK"() -> (w5320:refnum<vi>)
                n2618 = call "TestExec.Health Indicator State Controller.vi"("Go to Details"=w5317, "Errors Cntr"=w5318, "Warnings Cntr"=w5319, "Health Bool"=w5320) -> ()  [unwired: 8 in]
              }
            }
            n2619 = local write "Mode"(u16 0) -> ()
            n2620 = property on="Fail Cnt" class="DigNum (strict)"("NumText.BGColor"=w5315) -> ()  [unwired: 2 in, 2 out]
            n2621 = property on="Error Cnt" class="DigNum (strict)"("NumText.BGColor"=w5315) -> ()  [unwired: 2 in, 2 out]
            n2622 = property on="Status" class="Str"("Text.BGColor"=u32 13816530) -> ()  [unwired: 2 in, 2 out]
            n2623 = property on="Yield%" class="DigNum (strict)"("NumText.BGColor"=w5315) -> ()  [unwired: 2 in, 2 out]
            n2624 = property on="Abort Cnt" class="DigNum (strict)"("NumText.BGColor"=u32 16448250) -> ()  [unwired: 2 in, 2 out]
          }
          frame #4 {
            # "Wait for TCP-IP to send Exit to Child"
            n2625 = call <vilib>:"Time.Inline Delay.vi"("Wait(ms)"=u32 20) -> ("error out"=w5322:errorcluster)  [unwired: 9 in, 1 out]
            n2626 = call <vilib>:"Q.Enqueue Exit.vi"("Q Name"="TCP-IP_TE" ("Control Q Name"), "Error In"=w5322) -> ("error out"=w5324:errorcluster)  [unwired: 8 in, 1 out]
          }
        }
        n2627 = call <vilib>:"Module.Destructor.vi"("error in"=w5284, "Sys"=w5283) -> ("error out"=w5287:errorcluster)  [unwired: 9 in]
      }
    }
  }
  n2628 = while "Event Loop" {
    tunnel: w4 -> [w5328]
    stop <- w5329 stop-if-true
    n2629 = Unbundle By Name(w5328) -> ("Stop.Ref"=w5327:refnum<event-registration>, "Main Q"=w5326:refnum<queue>)
    n2630 = event shown="[7] \"Sync Now\": Value Change" {
      selector: w5327 -> [_ _ _ _ _ _ _ _ _ _ _ _ _ _ _ _ _ _ _ _ _ _ _ _ _ _ _ _ _ _ _ _ _ _ _ _ _ _ _ _ _ _ _ _ _ _ _ _ _]
      dyn-events: _ -> [_ _ _ _ _ _ _ _ _ _ _ _ _ _ _ _ _ _ _ _ _ _ _ _ _ _ _ _ _ _ _ _ _ _ _ _ _ _ _ _ _ _ _ _ _ _ _ _ _]
      timeout: 500 -> [_ _ _ _ _ _ _ _ _ _ _ _ _ _ _ _ _ _ _ _ _ _ _ _ _ _ _ _ _ _ _ _ _ _ _ _ _ _ _ _ _ _ _ _ _ _ _ _ _]
      tunnel: [w5332 _ _ w5350 _ _ _ _ _ _ _ _ _ _ _ _ _ _ _ _ _ _ _ _ _ _ TRUE _ _ _ _ _ _ _ _ _ _ _ _ _ _ _ _ _ _ _ _ _ _] -> w5329
      tunnel: w5328 -> [w5331 _ _ w5348 _ _ _ _ _ _ _ _ _ _ _ _ _ w5468 _ _ _ _ _ _ _ _ _ _ _ _ _ _ _ _ _ _ _ _ _ _ _ _ _ _ _ _ w5567 _ _]
      tunnel: w5326 -> [w5334 w5344 _ w5349 w5418 _ _ w5440 w5445 w5446 w5448 _ w5453 w5455 w5460 _ _ _ _ w5473 _ w5480 w5482 w5486 w5490 w5492 _ w5495 w5503 w5520 w5534 _ _ _ w5539 w5542 w5544 _ w5546 w5554 w5555 w5558 w5560 _ _ w5565 _ _ _]
      event Panel Close? {
        n2631 = event-data() -> ()  [unwired: 1 in, 4 out]
        n2632 = Unbundle By Name(w5331) -> ("Cfg.Is Child?"=w5330:bool)
        n2633 = case shown="True" w5330 {
          tunnel: w5334 -> [w5337 w5340]
          tunnel: [TRUE TRUE] -> w5333
          tunnel: [TRUE FALSE] -> w5332
          tunnel: [_ w5338] -> _
          frame False {
            # "Parent - Exit"
            n2634 = call <vilib>:"Q.Enqueue Exit.vi"("Q In"=w5337) -> ()  [unwired: 9 in, 2 out]
          }
          frame True {
            # "Child - Hide Panel and if was \nin a subpanel, return to subpanel."
            n2635 = call <vilib>:"Module.Window, Q Task.vi"("Action"=Window.Task,_Action."Return to SubPanel()", "Q In"=w5340) -> ("error out"=w5338:errorcluster)  [unwired: 8 in, 1 out]
          }
        }
        n2636 = event-data("Discard?"=w5333) -> ()  [unwired: 1 in, 1 out]
      }
      event Panel Resize {
        n2637 = event-data() -> ()  [unwired: 1 in, 8 out]
        n2638 = call <vilib>:"Module.Window, Q Task.vi"("Action"=Window.Task,_Action."Resize()", "Q In"=w5344) -> ()  [unwired: 8 in, 2 out]
      }
      event "Leave Maint": Value Change {
        n2639 = event-data() -> ()  [unwired: 1 in, 6 out]
        n2640 = local write "Main Tab"(0) -> ()
      }
      event Menu Selection (User) {
        n2641 = event-data() -> ("MenuRef"=w5346:refnum<k9>, "ItemTag"=w5347:string)  [unwired: 1 in, 5 out]
        n2642 = case shown="\"File Sync\"" w5347 {
          selector: w5347 -> [w5353 _ _ _ _ w5387 _ _ _ _ _ _ _ _ _ _ _]
          tunnel: [_ TRUE _ _ _ _ _ _ _ _ _ _ _ _ _ _ _] -> w5350
          tunnel: w5349 -> [w5352 w5374 _ w5381 _ w5391 w5393 w5395 w5397 w5399 w5403 _ w5408 w5410 w5412 w5414 w5417]
          tunnel: [_ _ w5378 _ _ _ _ _ _ _ _ _ _ _ _ _ _] -> _
          tunnel: w5348 -> [w5355 _ _ _ w5385 _ _ _ _ _ _ _ _ _ _ _ _]
          tunnel: w5346 -> [_ _ _ _ _ w5388 _ _ _ _ _ _ _ _ _ _ _]
          frame Default {
            n2643 = Match Pattern(string=w5353, regular expression="_") -> (before substring=w5351:string)  [unwired: 1 in, 3 out]
            n2644 = case shown="\"Data\"" w5351 {
              tunnel: w5355 -> [_ _ _ w5369]
              tunnel: w5353 -> [w5358 w5364 _ w5368]
              tunnel: w5352 -> [w5361 w5367 _ _]
              frame "Data" {
                n2645 = Match Pattern(string=w5358, regular expression="^Data_") -> (after substring=w5356:string)  [unwired: 1 in, 3 out]
                n2646 = To Variant(anything=w5356) -> (Variant=w5360:variant)
                n2647 = call <vilib>:"Q.Enqueue Task.vi"("Data1"=w5360, "Task Name"="Data - Open Folder", "Q In"=w5361) -> ()  [unwired: 7 in, 2 out]
              }
              frame "Config" {
                n2648 = Match Pattern(string=w5364, regular expression="^Config_") -> (after substring=w5362:string)  [unwired: 1 in, 3 out]
                n2649 = To Variant(anything=w5362) -> (Variant=w5366:variant)
                n2650 = call <vilib>:"Q.Enqueue Task.vi"("Data1"=w5366, "Task Name"="Config - Open Folder", "Q In"=w5367) -> ()  [unwired: 7 in, 2 out]
              }
              frame Default {
              }
              frame "Manuals" {
                n2651 = Unbundle By Name(w5369) -> ("Docs.Tags"=w5371:string[], "Docs.Paths"=w5370:path[])
                n2652 = call <vilib>:"Menu.Help, Open User Manual Items.vi"("Menu Tag Selection"=w5368, "Paths"=w5370, "Tags"=w5371) -> ()  [unwired: 8 in, 1 out]
              }
            }
          }
          frame "Exit" {
            n2653 = call <vilib>:"Q.Enqueue Exit.vi"("Q In"=w5374) -> ()  [unwired: 9 in, 2 out]
            n2654 = for {
              N: 10 -> [_]
              n2655 = call "Abort.Send Abort or Done Notificaiton.vi"("Abort(T)/Done(F)"=TRUE) -> ()  [unwired: 10 in, 1 out]
              n2656 = Wait (ms)(milliseconds to wait=u32 10) -> ()  [unwired: 1 out]
            }
            n2657 = local write "Abort Flag"(TRUE ("Abort Flag")) -> ()
          }
          frame "Event Log" {
            n2658 = call <vilib>:"Event Log.Show.vi"() -> ("error out"=w5378:errorcluster)  [unwired: 11 in]
          }
          frame "Reset" {
            n2659 = call <vilib>:"Q.Enqueue Reset.vi"("Q In"=w5381) -> ()  [unwired: 9 in, 2 out]
            n2660 = for {
              N: 10 -> [_]
              n2661 = call "Abort.Send Abort or Done Notificaiton.vi"("Abort(T)/Done(F)"=TRUE) -> ()  [unwired: 10 in, 1 out]
              n2662 = Wait (ms)(milliseconds to wait=u32 10) -> ()  [unwired: 1 out]
            }
            n2663 = local write "Abort Flag"(TRUE ("Abort Flag")) -> ()
          }
          frame "Help.About" {
            n2664 = Unbundle By Name(w5385) -> ("SW Rev"=w5384:T32)
            n2665 = call <vilib>:"Help.About.vi"("SW Version"=w5384) -> ()  [unwired: 11 in]
          }
